vi "Remove Shared Resource.vi"(8 "error in (no error)":errorcluster, 10 "RID":string, 11 "Controller in":refnum<class "Controller.lvclass">) -> (0 "error out":errorcluster, 3 "Controller out":refnum<class "Controller.lvclass">)   [LabVIEW 2013, in "SET Project Editor.lvlib" / "Controller.lvclass"]
uses:
  Controller.lvclass
  Controller.lvclass/Controller.ctl
  SET Project Data/Project Data Class/Project Data.lvclass
  SET Project Data/VI Class/VI Data.lvclass
  SET Project Data/Control Classes/GObject/GObject.lvclass/GObject.ctl
  <vilib>/ActorFramework/Message Enqueuer/Message Enqueuer.lvclass/Message Enqueuer.ctl
  SET Project Data/Control Classes/GObject/Read Items.vi
  <vilib>/ActorFramework/Message Enqueuer/Enqueue.vi
  SET Project Data/Control Classes/GObject/Read UID.vi
  <vilib>/ActorFramework/Message Priority Queue/Priority Enqueue.vi
  SET Project Data/Resource Data Class/Resource Data.lvclass
  UI View Messages/UI Refresh Data Msg/UI Refresh Data Msg.lvclass
  SET Project Data/Control Classes/GObject/GObject.lvclass
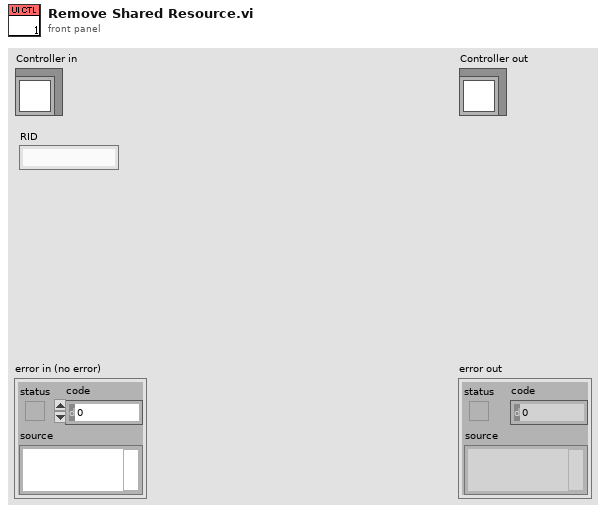
[diagram p1: front panel]
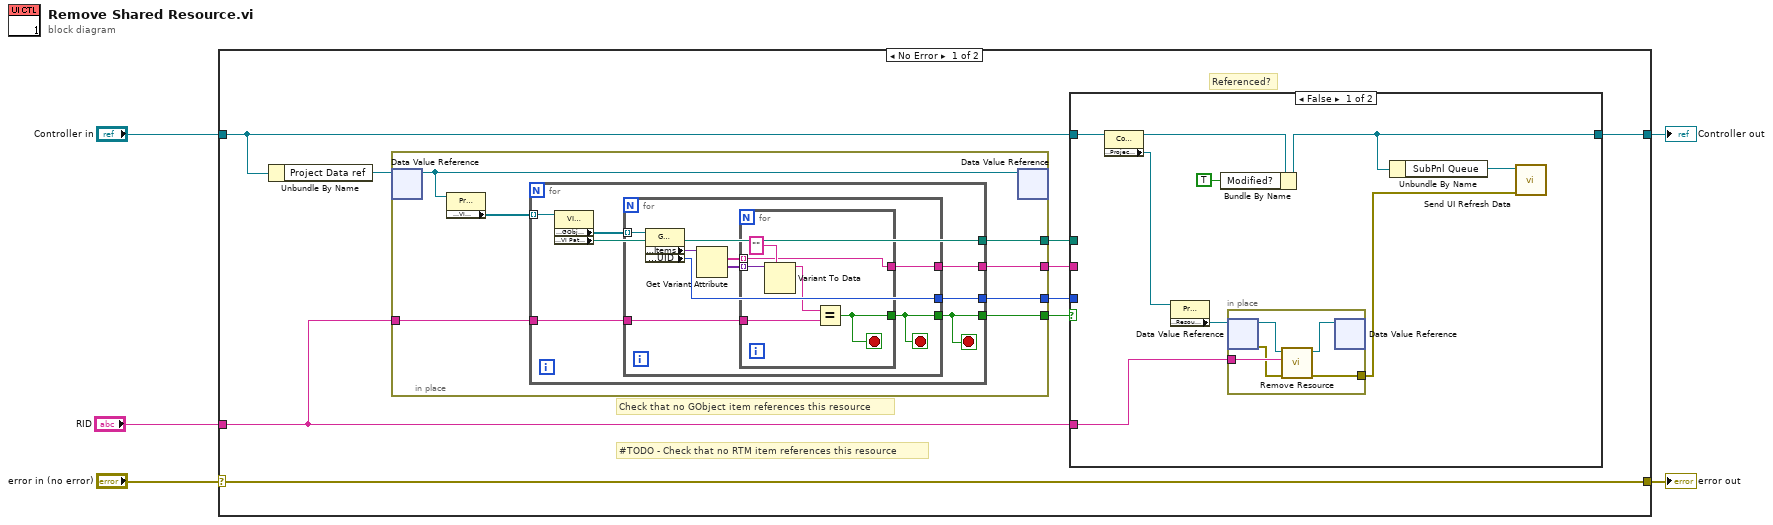
[diagram p0: block diagram]
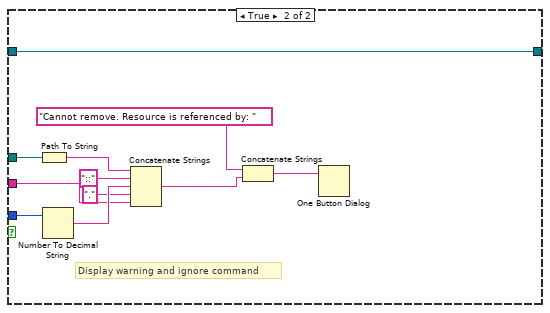
[diagram p2: hidden frame]
diagram:
  n1 = case shown="No Error" "error in (no error)" {
    selector: "error in (no error)" -> [w14 w69]
    tunnel: [w14 w69] -> w4
    tunnel: [w11 w68] -> w2
    tunnel: "Controller in" -> [w12 w68]
    tunnel: "RID" -> [w6 _]
    frame No Error {
      # "#TODO - Check that no RTM item references this resource"
      # "Check that no GObject item references this resource"
      # "Referenced?"
      n2 = Unbundle By Name(w12) -> ("Project Data ref"=w13:refnum<data-value>)
      n3 = in-place {
        in-place-border: w6 -> [w45]
        in-place-border: [w43] -> w10
        in-place-border: [w42] -> w9
        in-place-border: [w41] -> w8
        in-place-border: [w40] -> w7
        n4 = in-place-dvr #1(w13) -> (w44:refnum<class "Project Data.lvclass">)  [unwired: 1 out]
        n5 = property class="Project Data.lvclass"(reference=w44) -> ("Properties:VI Table"=w46:refnum<class "VI Data.lvclass">[])  [unwired: 1 in, 2 out]
        n6 = for {
          tunnel: w46 -> [w53] mode=indexing
          tunnel: w45 -> [w51]
          tunnel: [w50] -> w43
          tunnel: [w49] -> w42
          tunnel: [w48] -> w41
          tunnel: [w47] -> w40
          stop <- w50 stop-if-true
          n7 = property class="VI Data.lvclass"(reference=w53) -> ("Properties:GObjects"=w52:refnum<class "GObject.lvclass">[], "Properties:VI Path (Relative)"=w47:path)  [unwired: 1 in, 2 out]
          n8 = for {
            tunnel: w52 -> [w61] mode=indexing
            tunnel: w51 -> [w57]
            tunnel: [w56] -> w50
            tunnel: [w55] -> w49
            tunnel: [w54] -> w48
            stop <- w56 stop-if-true
            n9 = property class="GObject.lvclass"(reference=w61) -> ("Properties:Items"=w60:variant, "Properties:UID"=w54:i32)  [unwired: 1 in, 2 out]
            n10 = Get Variant Attribute(Variant=w60) -> (names=w59:string[], values=w58:variant[])  [unwired: 3 in, 2 out]
            n11 = for {
              tunnel: w59 -> [w62] mode=indexing
              tunnel: w58 -> [w67] mode=indexing
              tunnel: w57 -> [w65]
              tunnel: [w64] -> w56
              tunnel: [w62] -> w55
              stop <- w64 stop-if-true
              n12 = Variant To Data(type="", Variant=w67) -> (data=w63:string)  [unwired: 1 in, 1 out]
              n13 = Equal?(x=w63, y=w65) -> (x = y?=w64:bool)
            }
          }
        }
        n14 = in-place-dvr #1(w44) -> ()  [unwired: 2 out]
      }
      n15 = case shown="False" w10 {
        tunnel: w12 -> [w23 w39]
        tunnel: [w16 w39] -> w11
        tunnel: w9 -> [_ w32]
        tunnel: w8 -> [_ w37]
        tunnel: w7 -> [_ w38]
        tunnel: w6 -> [w20 _]
        frame False {
          n16 = property class="Controller.lvclass"(reference=w23) -> (reference out=w17:refnum<class "Controller.lvclass">, "Properties:Project Data ref"=w22:refnum<data-value>)  [unwired: 1 in, 1 out]
          n17 = property class="Project Data.lvclass"(reference=w22) -> ("Properties:Resource Data ref"=w21:refnum<data-value>)  [unwired: 1 in, 2 out]
          n18 = Bundle By Name(cluster=w17, "Modified?"=TRUE) -> (w16:refnum<class "Controller.lvclass">)
          n19 = in-place {
            in-place-border: w20 -> [w26]
            in-place-border: [w24] -> w18
            n20 = in-place-dvr #2(w21) -> (w28:refnum<class "Resource Data.lvclass">, w25:errorcluster)
            n21 = call "Remove Resource.vi"("error in (no error)"=w25, "RID"=w26, "LangFile in"=w28) -> ("error out"=w24:errorcluster, "LangFile out"=w27:refnum<class "Resource Data.lvclass">)  [unwired: 7 in]
            n22 = in-place-dvr #2(w27) -> ()  [unwired: 2 out]
          }
          n23 = Unbundle By Name(w16) -> ("SubPnl Queue"=w19:refnum<class "Message Enqueuer.lvclass">)
          n24 = call "Send UI Refresh Data.vi"("error in (no error)"=w18, "Message Enqueuer"=w19) -> ()  [unwired: 8 in, 2 out]
        }
        frame True {
          # "Display warning and ignore command"
          n25 = Path To String(path=w38) -> (string=w36:string)
          n26 = Number To Decimal String(number=w37) -> (decimal integer string=w34:string)  [unwired: 1 in]
          n27 = Concatenate Strings(w36, "::" ("string"), w34, "." ("string"), w32) -> (w30:string)
          n28 = Concatenate Strings("Cannot remove. Resource is referenced by: " ("string"), w30) -> (w29:string)
          n29 = One Button Dialog(message=w29) -> ()  [unwired: 1 in, 1 out]
        }
      }
    }
    frame Error {
    }
  }
  "error out" <- w4
  "Controller out" <- w2
